vi "Read Test Data (AC Phase B Program Mode).vi"(0 "VISA resource name":refnum<visa-resource-name>, 11 "error in (no error)":errorcluster) -> (4 "VISA resource name out":refnum<visa-resource-name>, 6 "Test Meter Data Output":T1 {"Timer (s)" format="%.1f"; "Frequency (Hz)" format="%.1f"; "Voltage (V)" format="%.1f"; "RMS Current (A)" format="%.3f"; "Power (W)" format="%.1f"; "Peak Current (A)" format="%.1f"; "Power Factor" format="%.3f"; "Power Resistive (VAR)" format="%.1g"; "Crest Factor" format="%.2f"; "Power Apparent (VA)" format="%.1g"}, 15 "error out":errorcluster)   [LabVIEW 2016, in "APT 300XAC Series.lvlib"]
doc: "Reads the Program mode <B>active data being displayed on the LCD display</B> while the test is in process. It also gives the last data taken when the test sequence completed. \n\nIn Program Mode the output data cluster has the following data.\n\n1. Memory\n2. Step\n3. Timer (s)\n4. Frequency (Hz)\n5. Voltage (V)\n6. RMS Current (A)\n7. Power (W)\n8. Power Resistive\n9. Peak Current (A)\n10. Crest Factor\n11. Power Factor\n12. Power Apparent (VA)\n13. Status"
uses:
  APT 300XAC Series.lvlib
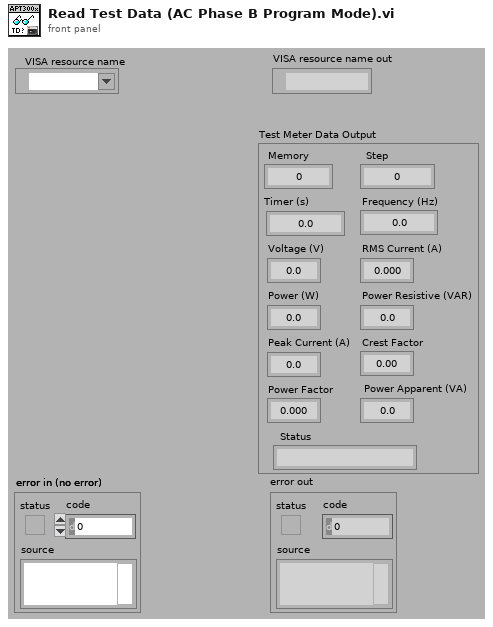
[diagram p1: front panel]
types:
  T1 = cluster{"Memory":i32, "Step":i32, "Timer (s)":dbl, "Frequency (Hz)":dbl, "Voltage (V)":dbl, "RMS Current (A)":dbl, "Power (W)":dbl, "Peak Current (A)":dbl, "Power Factor":dbl, "Status":string, "Power Resistive (VAR)":dbl, "Crest Factor":dbl, "Power Apparent (VA)":dbl}
  T2 = cluster{"Memory":i32, "Step":i32, "Timer":dbl, "Frequency":dbl, "Volt":dbl, "Current":dbl, "Power":dbl, "Peak Current":dbl, "Power Factor":dbl, "Status":string, "Power Resistive":dbl, "Crest Factor":dbl, "Power Apparent":dbl}
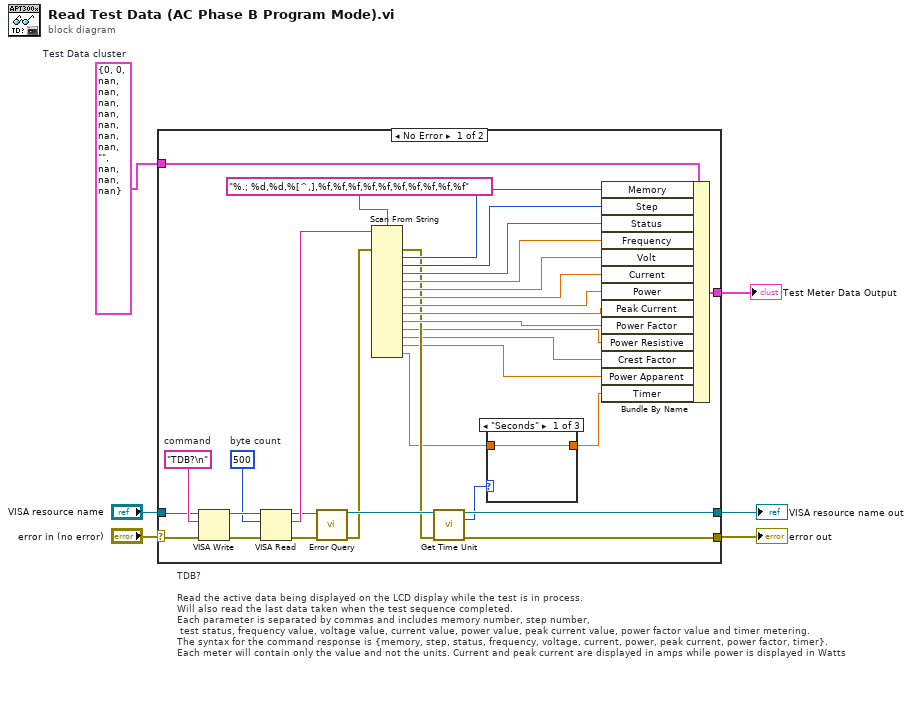
[diagram p0: block diagram]
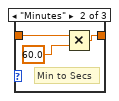
[diagram p2: hidden frame]
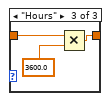
[diagram p3: hidden frame]
diagram:
  w2 = T2 {"Memory"=0, "Step"=0, "Timer"=nan, "Frequency"=nan, "Volt"=nan, "Current"=nan, "Power"=nan, "Peak Current"=nan, "Power Factor"=nan, "Status"="", "Power Resistive"=nan, "Crest Factor"=nan, "Power Apparent"=nan}  # Test Data cluster
  # "TDB?\n\nRead the active data being displayed on the LCD display while the test is in process. \nWill also read the last data taken when the test sequence completed. \nEach parameter is separated by commas and includes memory number, step number,\n test status, frequency value, voltage value, current value, power value, peak current value, power factor value and timer metering. \nThe syntax for the command response is {memory, step, status, frequency, voltage, current, power, peak current, power factor, timer}. \nEach meter will contain only the value and not the units. Current and peak current are displayed in amps while power is displayed in Watts"
  n1 = case shown="No Error" "error in (no error)" {
    selector: "error in (no error)" -> [w31 w47]
    tunnel: "VISA resource name" -> [w32 w48]
    tunnel: [w29 w48] -> w4
    tunnel: [w30 w47] -> w3
    tunnel: [w35 w46] -> w1
    tunnel: w2 -> [w34 w46]
    frame No Error {
      w33 = "TDB?\n"  # command
      w36 = u32 500  # byte count
      n2 = VISA Write(VISA resource name=w32, write buffer=w33, error in (no error)=w31) -> (VISA resource name out=w38:refnum<visa-resource-name>, error out=w37:errorcluster)  [unwired: 1 out]
      n3 = VISA Read(VISA resource name=w38, byte count=w36, error in (no error)=w37) -> (VISA resource name out=w16:refnum<visa-resource-name>, read buffer=w17:string, error out=w15:errorcluster)  [unwired: 1 out]
      n4 = call "Error Query.vi"("VISA resource name"=w16, "error in (no error)"=w15) -> ("VISA resource name out"=w14:refnum<visa-resource-name>, "error out"=w13:errorcluster)  [unwired: 10 in, 2 out]
      n5 = Scan From String(format string="%.; %d,%d,%[^,],%f,%f,%f,%f,%f,%f,%f,%f,%f,%f", input string=w17, error in=w13) -> (error out=w12:errorcluster, output 1=w26:i32, output 2=w25:i32, output 3=w24:string, output 4=w23:dbl, output 5=w22:dbl, output 6=w21:dbl, output 7=w20:dbl, output 8=w19:dbl, output 9=w18:dbl, output 10=w10:dbl, output 11=w9:dbl, output 12=w8:dbl, output 13=w11:dbl)  [unwired: 14 in, 2 out]
      n6 = call "Get Time Unit.vi"("VISA resource name"=w14, "error in (no error)"=w12) -> ("VISA resource name out"=w29:refnum<visa-resource-name>, "Time Unit"=w28:enum16{"Seconds", "Minutes", "Hours"}, "error out"=w30:errorcluster)  [unwired: 11 in]
      n7 = case shown="\"Seconds\"" w28 {
        tunnel: [w39 w41 w44] -> w7
        tunnel: w11 -> [w39 w40 w43]
        frame "Seconds" {
        }
        frame "Minutes" {
          # "Min to Secs"
          n8 = Multiply(x=w40, y=60.0) -> (x*y=w41:dbl)
        }
        frame "Hours" {
          n9 = Multiply(x=w43, y=3600.0) -> (x*y=w44:dbl)
        }
      }
      n10 = Bundle By Name(cluster=w34, "Memory"=w26, "Step"=w25, "Status"=w24, "Frequency"=w23, "Volt"=w22, "Current"=w21, "Power"=w20, "Peak Current"=w19, "Power Factor"=w18, "Power Resistive"=w10, "Crest Factor"=w9, "Power Apparent"=w8, "Timer"=w7) -> (w35:T2)
    }
    frame Error {
    }
  }
  "VISA resource name out" <- w4
  "error out" <- w3
  "Test Meter Data Output" <- w1
